vi "Get Path Regex.vi"(8 "error in (no error)":errorcluster, 11 "Submission API in":refnum<class "User Submissions API.lvclass">) -> (0 "error out":errorcluster, 2 "Path Regex":string, 3 "Submission API out":refnum<class "User Submissions API.lvclass">)   [LabVIEW 2020, in "Summer of LabVIEW.lvlib" / "User Submissions API.lvclass"]
uses:
  User Submissions API.lvclass
  User Submissions API.lvclass/User Submissions API.ctl
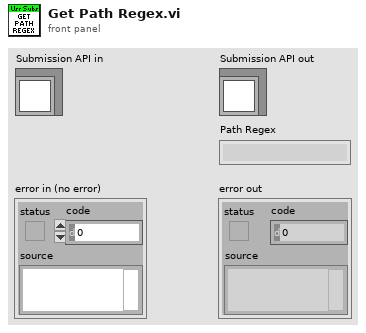
[diagram p1: front panel]
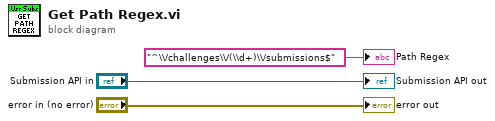
[diagram p0: block diagram]
diagram:
  "error out" <- "error in (no error)"
  "Submission API out" <- "Submission API in"
  "Path Regex" <- "^\\/challenges\\/(\\d+)\\/submissions$" ("Path Regex")
